vi "Encoding Message from GUI.vi"(8 "Data":string, 9 "Message":string, 10 "uS/GD ID":string, 11 "uService Template in":refnum<class "Kasli Writer.lvclass">) -> (2 "Variant":variant, 3 "uService Template out":refnum<class "Kasli Writer.lvclass">)   [LabVIEW 2020, in "CIRCUS_uServices.lvlib" / "Kasli Listener and Writer.lvlib" / "Kasli Writer.lvclass"]
uses:
  Kasli Writer.lvclass
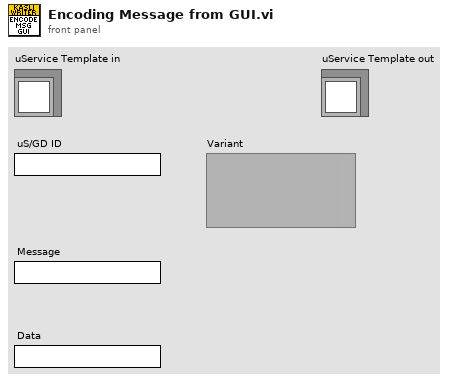
[diagram p1: front panel]
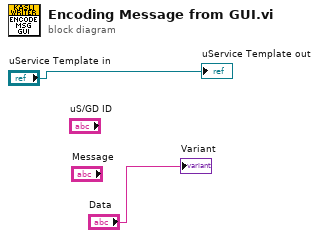
[diagram p0: block diagram]
diagram:
  "Variant" <- "Data"
  "uService Template out" <- "uService Template in"
